vi "Player Get Snake Element.vi"(8 "error in (no error)":errorcluster, 10 "Index":i32, 11 "Player in":refnum<class "Player.lvclass">) -> (0 "error out":errorcluster, 2 "Snake":refnum<class "Snake.lvclass">, 3 "Player out":refnum<class "Player.lvclass">)   [LabVIEW 2019, in "Player.lvclass"]
uses:
  Player.lvclass
  Snake/Snake.lvclass
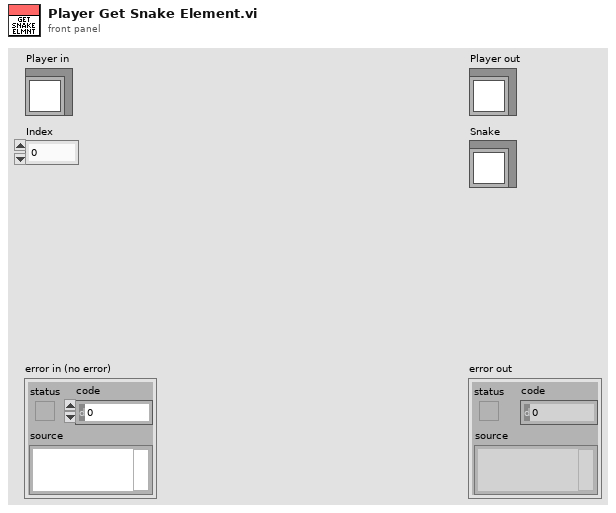
[diagram p1: front panel]
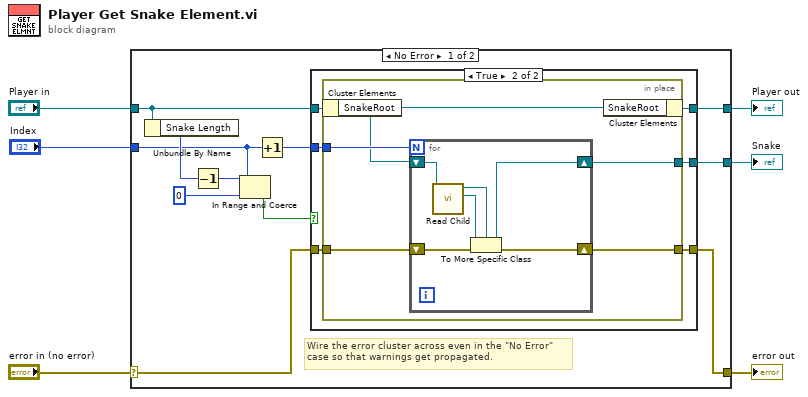
[diagram p0: block diagram]
diagram:
  n1 = case shown="No Error" "error in (no error)" {
    selector: "error in (no error)" -> [w9 w37]
    tunnel: [w8 w37] -> w2
    tunnel: [w10 w38] -> w4
    tunnel: "Player in" -> [w11 w38]
    tunnel: "Index" -> [w13 _]
    tunnel: [w7 _] -> w1
    frame No Error {
      # "Wire the error cluster across even in the \"No Error\"\ncase so that warnings get propagated."
      n2 = Unbundle By Name(w11) -> ("Snake Length"=w16:i32)
      n3 = Decrement(x=w16) -> (x-1=w15:i32)
      n4 = In Range and Coerce(upper limit=w15, x=w13, lower limit=0) -> (In Range?=w14:bool)  [unwired: 1 out]
      n5 = Increment(x=w13) -> (x+1=w12:i32)
      n6 = case shown="True" w14 {
        tunnel: w12 -> [_ w25]
        tunnel: w11 -> [w19 w24]
        tunnel: [w19 w23] -> w10
        tunnel: w9 -> [w18 w22]
        tunnel: [w18 w21] -> w8
        tunnel: [_ w20] -> w7
        frame False {
        }
        frame True {
          n7 = in-place {
            in-place-border: w25 -> [w30]
            in-place-border: w22 -> [w28]
            in-place-border: [w27] -> w21
            in-place-border: [w26] -> w20
            n8 = in-place-cluster #1(w24) -> ("SnakeRoot"=w29:refnum<class "Snake.lvclass">)
            n9 = for {
              N: w30 -> [_]
              shift-right: [w33] -> w26
              shift-left: w29 -> [w36]
              shift-right: [w31] -> w27
              shift-left: w28 -> [w32]
              n10 = call-dynamic "Read Child.vi"("Snake in"=w36) -> ("Child"=w35:refnum<class>, "Snake out"=w34:refnum<class "Snake.lvclass">)  [unwired: 8 in, 1 out]
              n11 = To More Specific Class(target class=w34, reference=w35, error in=w32) -> (specific class reference=w33:refnum<class "Snake.lvclass">, error out=w31:errorcluster)
            }
            n12 = in-place-cluster #1("SnakeRoot"=w29) -> (w23:refnum<class "Player.lvclass">)
          }
        }
      }
    }
    frame Error {
    }
  }
  "error out" <- w2
  "Player out" <- w4
  "Snake" <- w1
